vi "Read CAN.vi"() -> ()   [LabVIEW 2015]
uses:
  sbrio-2018/Formula Hybrid 2012 r1/Global Data.vi
panel:
  out "CAN Log Error":errorcluster
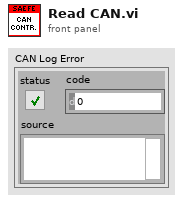
[diagram p1: front panel]
types:
  T1 = cluster{"read mode":enum16{"polling", "blocking"}, "write mode":enum16{"polling", "blocking"}}
  T2 = typedef "CANFrameControl.ctl" = cluster{"identifier":u32, "extended?":bool, "type":u8, "payload":u8[]}
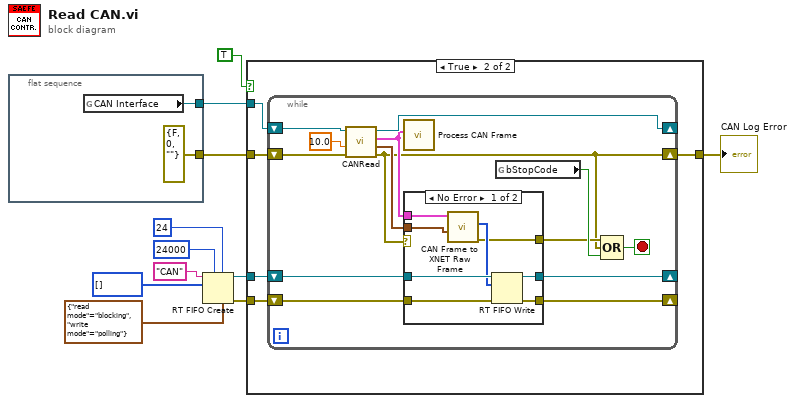
[diagram p0: block diagram]
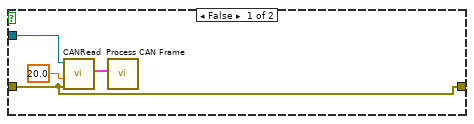
[diagram p2: hidden frame]
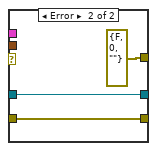
[diagram p3: hidden frame]
diagram:
  n1 = flat-sequence {
    tunnel: [errorcluster {"status"=FALSE, "code"=0, "source"=""} ("error out")] -> w5
    tunnel: [w12] -> w4
    frame #0 {
      n2 = global read "Global Data.vi" "CAN Interface"() -> (w12:refnum<k20>)
    }
  }
  n3 = RT FIFO Create(0:"CAN" ("name (unnamed)"), 1:u8[] [], 4:u32 24000 ("size (10)"), 6:u32 24 ("elements in array (1)"), 7:T1 {"read mode"=enum."blocking", "write mode"=enum."polling"} ("r/w modes (polling,polling)")) -> (8:w9:refnum<k33>, 11:w8:errorcluster)  [unwired: 3 in, 1 out]
  n4 = case shown="True" TRUE {
    tunnel: w4 -> [w17 w22]
    tunnel: w5 -> [w16 w21]
    tunnel: [w16 w20] -> w3
    tunnel: w9 -> [_ w19]
    tunnel: w8 -> [_ w18]
    frame False {
      n5 = call <vilib>:"CANRead.vi"("error in (no error)"=w16, "timeout (0 s)"=20.0, "interface object in"=w17) -> ("CAN frame"=w14:T2)  [unwired: 5 in, 3 out]
      n6 = call "Process CAN Frame.vi"("CAN frame"=w14) -> ()  [unwired: 11 in]
    }
    frame True {
      n7 = while {
        shift-right: [w36] -> _
        shift-left: w22 -> [w35]
        shift-right: [w23] -> w20
        shift-left: w21 -> [w33]
        shift-right: [w30] -> _
        shift-left: w19 -> [w32]
        shift-right: [w29] -> _
        shift-left: w18 -> [w31]
        stop <- w26 stop-if-true
        n8 = call <vilib>:"CANRead.vi"("error in (no error)"=w33, "timeout (0 s)"=10.0, "interface object in"=w35) -> ("error out"=w23:errorcluster, "timestamp"=w28:timestamp, "CAN frame"=w27:T2, "interface object out"=w36:refnum<k20>)  [unwired: 5 in]
        n9 = call "Process CAN Frame.vi"("CAN frame"=w27) -> ()  [unwired: 11 in]
        n10 = case shown="No Error" w23 {
          tunnel: w32 -> [w44 w47]
          tunnel: w31 -> [w43 w46]
          tunnel: [w42 w47] -> w30
          tunnel: [w41 w46] -> w29
          tunnel: w28 -> [w40 _]
          tunnel: w27 -> [w39 _]
          tunnel: [w37 errorcluster {"status"=FALSE, "code"=0, "source"=""} ("error out")] -> w24
          frame No Error {
            n11 = call "CAN Frame to XNET Raw Frame.vi"("timestamp"=w40, "CAN frame"=w39) -> ("error out"=w37:errorcluster, "Raw Frame"=w38:u8[])  [unwired: 8 in]
            n12 = RT FIFO Write(0:w44, 1:w38, 3:w43) -> (8:w42:refnum<k33>, 11:w41:errorcluster)  [unwired: 2 in, 2 out]
          }
          frame Error {
          }
        }
        n13 = global read "Global Data.vi" "bStopCode"() -> (w25:bool)
        n14 = Compound Arithmetic op=OR(w24, w23, w25) -> (w26:bool)
      }
    }
  }
  "CAN Log Error" <- w3
